vi "NanoSphereNew.vi"() -> ()   [LabVIEW 2011]
uses:
  <vilib>/Utility/file.llb/Write To Spreadsheet File (DBL).vi
  <vilib>/Utility/file.llb/Read From Spreadsheet File (DBL).vi
  <vilib>/Analysis/NI_AALBase.lvlib
panel:
  out "Current sensitivity 3":dbl
  out "Current sensitivity 2":dbl
  in  "stop":bool
  in  "stop 2":bool
  out "mean":dbl format="%0.2f"
  out "standard deviation":dbl format="%0.2f"
  out "XY Graph":cluster{"Y":dbl[], "Y":dbl[]}[](graph)
  in  "Angle":dbl
  in  "Max sensitivity":dbl
  out "data":dynamicdata(graph) caption="Current Data"
  in  "file path (dialog if empty)":path
  in  "Current sensitivity":dbl
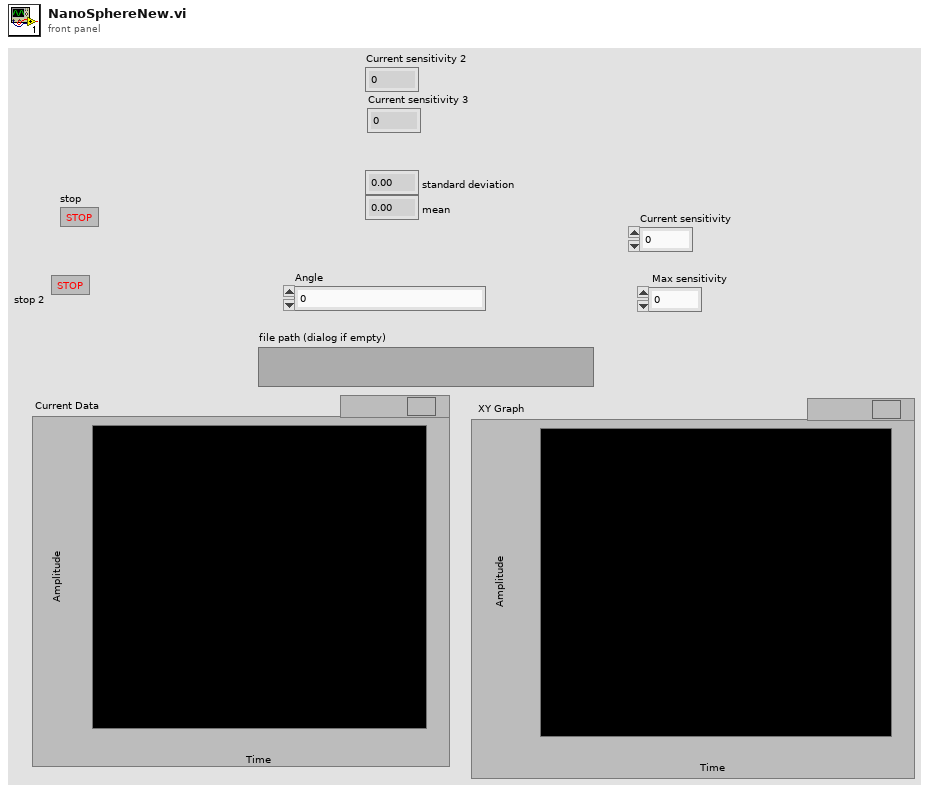
[diagram p1: front panel]
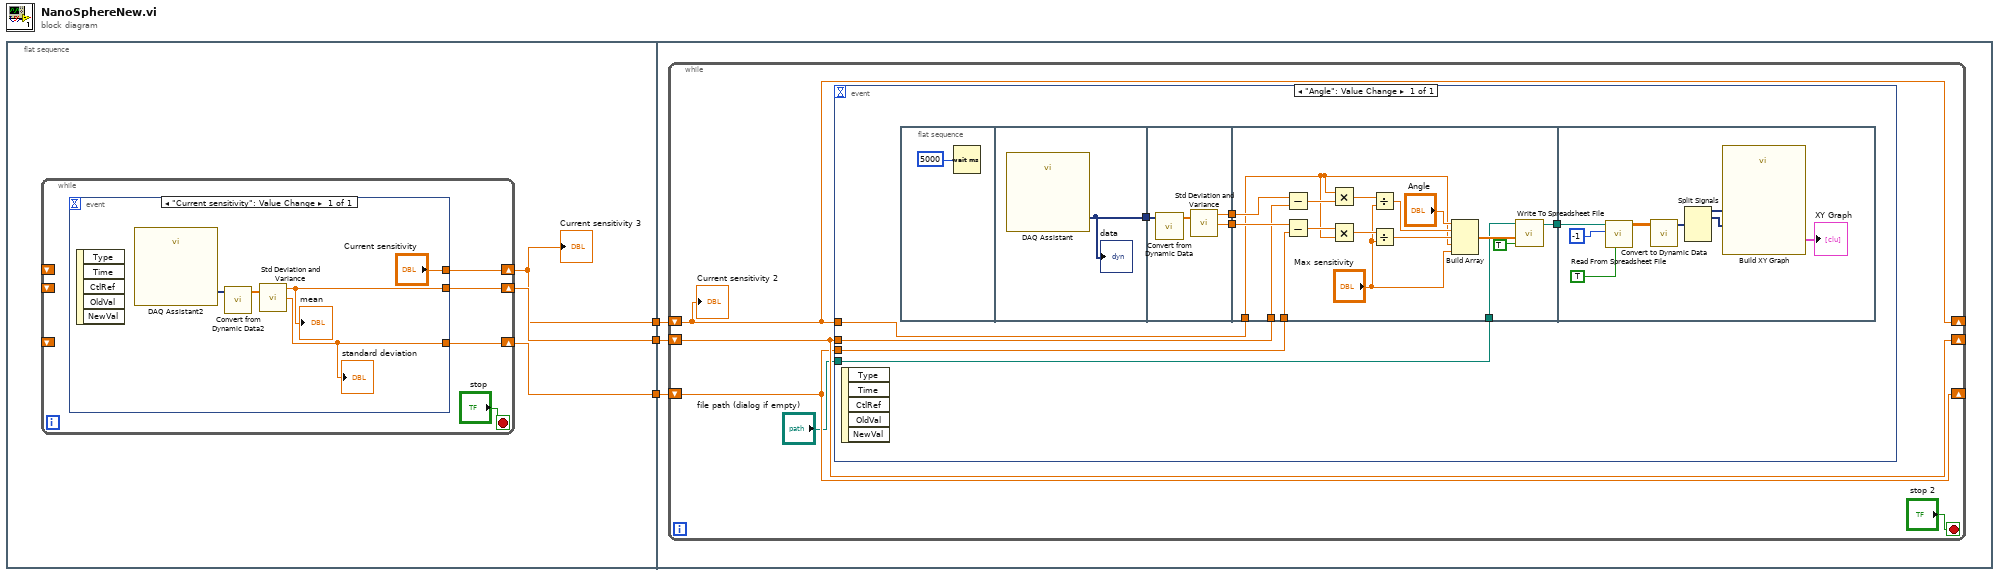
[diagram p0: block diagram]
diagram:
  n1 = flat-sequence {
    tunnel: [w6] -> w3
    tunnel: [w5] -> w2
    tunnel: [w4] -> w1
    tunnel: w3 -> [w18]
    tunnel: w2 -> [w17]
    tunnel: w1 -> [w16]
    frame #0 {
      n2 = while {
        shift-right: [w8] -> w4
        shift-left: _ -> [_]
        shift-right: [w10] -> w6
        shift-left: _ -> [_]
        shift-right: [w9] -> w5
        shift-left: _ -> [_]
        stop <- "stop" stop-if-true
        n3 = event shown="[0] \"Current sensitivity\": Value Change" {
          selector: _ -> [_]
          dyn-events: _ -> [_]
          timeout: _ -> [_]
          tunnel: [w13] -> w10
          tunnel: [w12] -> w9
          tunnel: ["Current sensitivity"] -> w8
          event "Current sensitivity": Value Change {
            n4 = event-data() -> ()  [unwired: 1 in, 5 out]
            n5 = call "DAQ Assistant2"() -> ("data"=w15:dynamicdata)  [unwired: 17 in, 2 out]
            n6 = call "Convert from Dynamic Data2"("Dynamic Data Type"=w15) -> ("Array"=w14:dbl[])  [unwired: 3 in]
            n7 = call <vilib>:"Std Deviation and Variance.vi"("X"=w14) -> ("mean"=w13:dbl, "standard deviation"=w12:dbl)  [unwired: 1 in, 1 out]
            "standard deviation" <- w12
            "mean" <- w13
          }
        }
      }
      "Current sensitivity 3" <- w4
    }
    frame #1 {
      n8 = while {
        shift-right: [w23] -> _
        shift-left: w16 -> [w23]
        shift-right: [w22] -> _
        shift-left: w18 -> [w22]
        shift-right: [w21] -> _
        shift-left: w17 -> [w21]
        stop <- "stop 2" stop-if-true
        n9 = event shown="[0] \"Angle\": Value Change" {
          selector: _ -> [_]
          dyn-events: _ -> [_]
          timeout: _ -> [_]
          tunnel: "file path (dialog if empty)" -> [w28]
          tunnel: w22 -> [w26]
          tunnel: w21 -> [w25]
          tunnel: w23 -> [w24]
          event "Angle": Value Change {
            n10 = event-data() -> ()  [unwired: 1 in, 5 out]
            n11 = flat-sequence {
              tunnel: [w33] -> w31
              tunnel: w31 -> [w37]
              tunnel: [w35] -> w30
              tunnel: [w34] -> w29
              tunnel: w30 -> [w44]
              tunnel: w29 -> [w42]
              tunnel: w28 -> [w53]
              tunnel: [w45] -> w27
              tunnel: w26 -> [w40]
              tunnel: w25 -> [w39]
              tunnel: w24 -> [w38]
              tunnel: w27 -> [w62]
              frame #0 {
                n12 = Wait (ms)(milliseconds to wait=u32 5000 ("millisecond timer value")) -> ()  [unwired: 1 out]
              }
              frame #1 {
                n13 = call "DAQ Assistant"() -> ("data"=w33:dynamicdata)  [unwired: 17 in, 2 out]
                "data" <- w33
              }
              frame #2 {
                n14 = call "Convert from Dynamic Data"("Dynamic Data Type"=w37) -> ("Array"=w36:dbl[])  [unwired: 3 in]
                n15 = call <vilib>:"Std Deviation and Variance.vi"("X"=w36) -> ("mean"=w35:dbl, "standard deviation"=w34:dbl)  [unwired: 1 in, 1 out]
              }
              frame #3 {
                n16 = Subtract(x=w44, y=w40) -> (x-y=w43:dbl)
                n17 = Subtract(x=w42, y=w39) -> (x-y=w41:dbl)
                n18 = Multiply(x=w38, y=w43) -> (x*y=w50:dbl)
                n19 = Multiply(x=w41, y=w38) -> (x*y=w48:dbl)
                n20 = Divide(x=w50, y="Max sensitivity") -> (x/y=w49:dbl)
                n21 = Divide(x=w48, y="Max sensitivity") -> (x/y=w47:dbl)
                n22 = Build Array("Angle", w49, w47, w38, "Max sensitivity") -> (w54:dbl[])
                n23 = call-poly <vilib>:"Write To Spreadsheet File.vi"("append to file? (new file:F)"=TRUE, "1D data"=w54, "file path (dialog if empty)"=w53) -> ("new file path (Not A Path if cancelled)"=w45:path)  [unwired: 5 in]
              }
              frame #4 {
                n24 = call-poly <vilib>:"Read From Spreadsheet File.vi"("transpose (no:F)"=TRUE, "number of rows (all:-1)"=-1, "file path (dialog if empty)"=w62) -> ("all rows"=w59:dbl[][])  [unwired: 4 in, 4 out]
                n25 = call "Convert to Dynamic Data"("2D Array"=w59) -> ("Dynamic Data Type"=w58:dynamicdata)  [unwired: 3 in]
                n26 = Split Signals(w58) -> (w56:dynamicdata, w55:dynamicdata)  [unwired: 5 in, 3 out]
                n27 = call "Build XY Graph"("Y Input"=w55, "X Input"=w56) -> ("XY Graph"=→"XY Graph":cluster{"Y":dbl[], "Y":dbl[]}[])  [unwired: 3 in, 6 out]
              }
            }
          }
        }
        "Current sensitivity 2" <- w23
      }
    }
  }
